vi "Generate NIPKG List.vi"() -> ()   [LabVIEW 2017]
uses:
  <vilib>/National Instruments/NIPM API (Beta)/_support/package attributes.ctl
  <vilib>/National Instruments/NIPM API (Beta)/NIPM_API.lvlib
  NIPKG Support/NIPKG SBOM Support.lvlib
panel:
  in  "stop":bool
  out "Current Package":T1={"Package Name"="", "Display name"="", "Version"="", "Display version"="", "Synopsis"="", "Description"="", "Maintainer"="", "Maintainer email address"="", "Category"="", "Homepage"="", "Release notes"="", "Depends"=[], "Recommends"=[], "Suggests"=[], "Conflicts"=[], "Provides"=[], "Replaces"=[], "Supplements"=[], "Enhances"=[], "Product"=FALSE, "User visible"=FALSE, "Installed size (KB)"=0, "Package filesize (bytes)"=0, "Architecture"="", "Agent"="file", "MD5Checksum"=""}
  out "Installed NI Packages":string[][](table)
  # "Retrieves list of all installed NIPKGs"
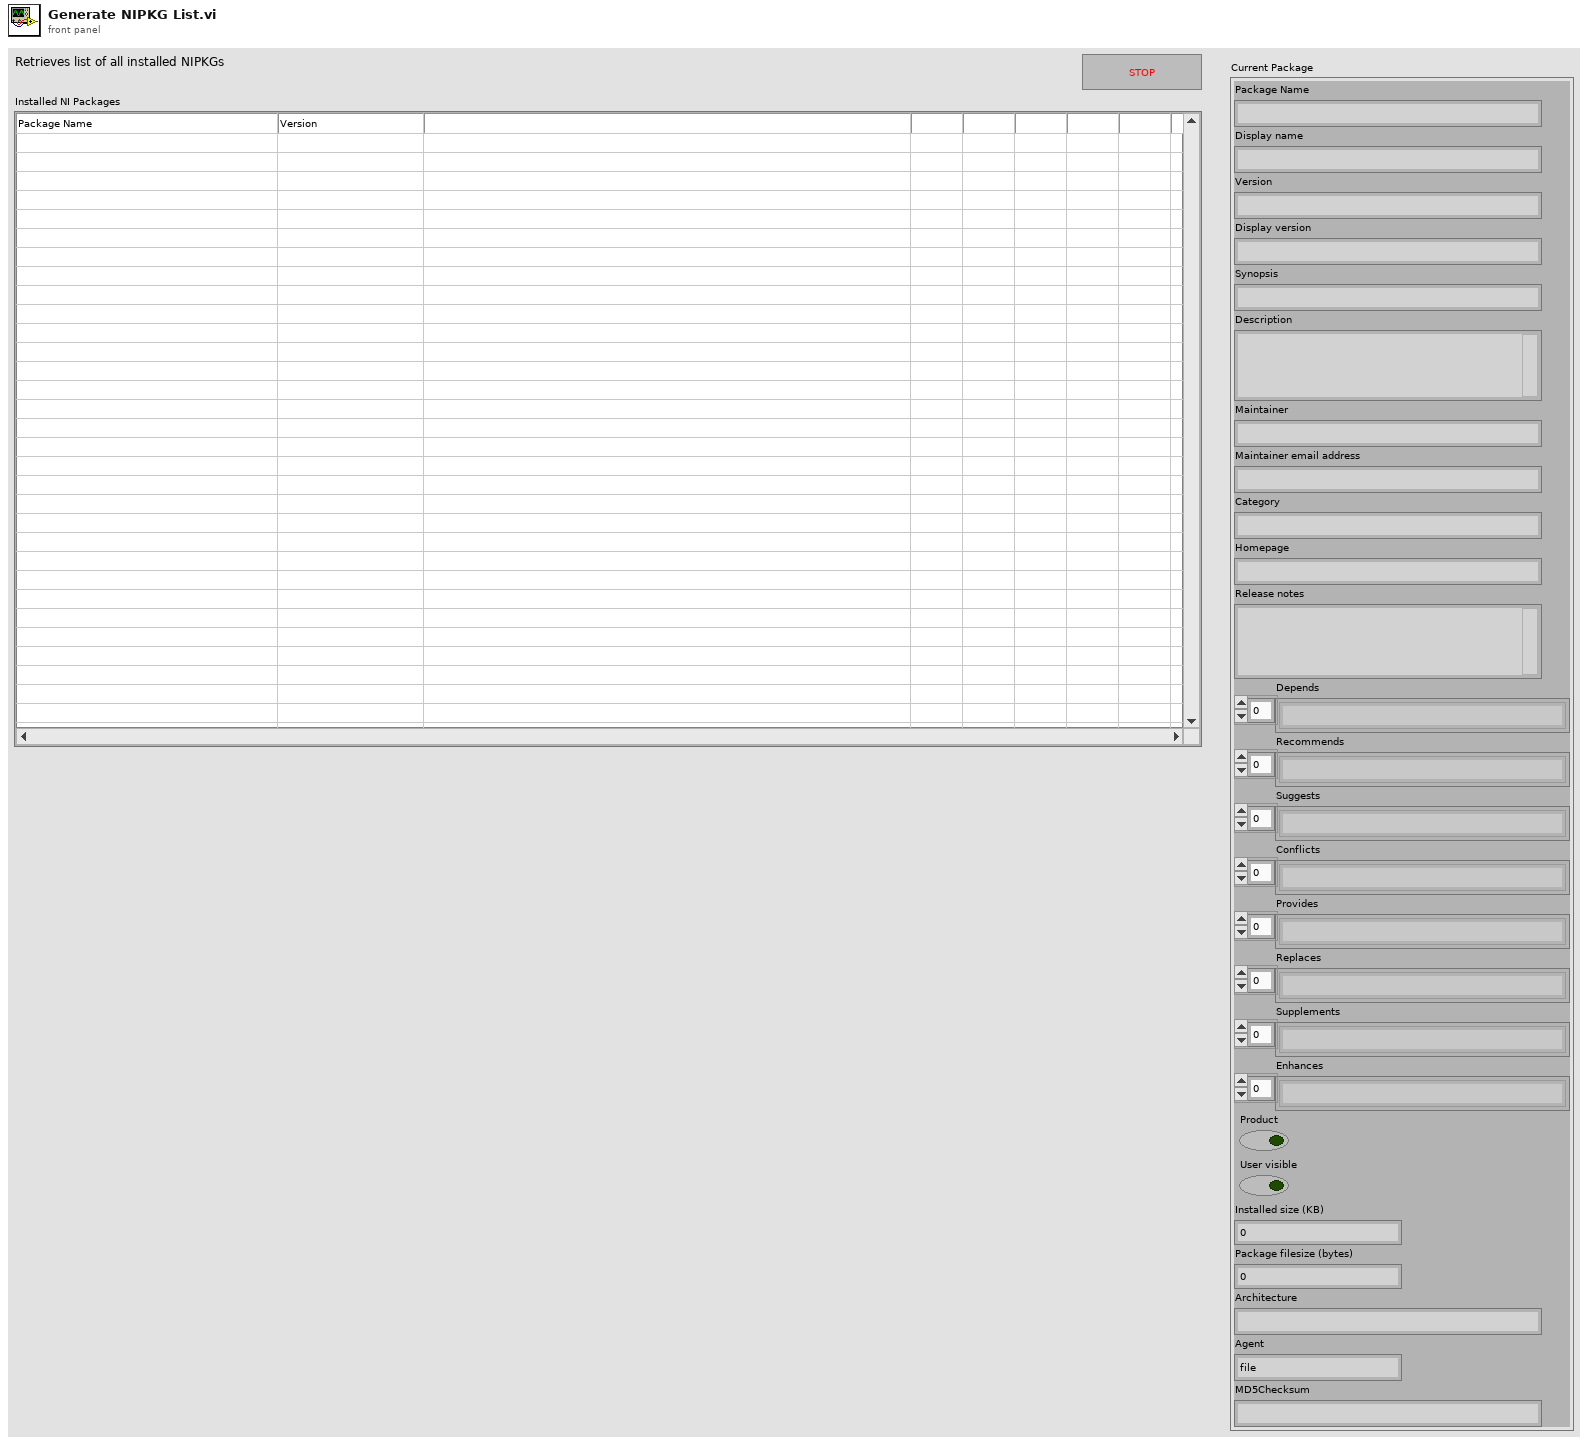
[diagram p1: front panel]
types:
  T1 = typedef "NIPM_API.lvlib/package attributes.ctl" = cluster{"Package Name":string, "Display name":string, "Version":string, "Display version":string, "Synopsis":string, "Description":string, "Maintainer":string, "Maintainer email address":string, "Category":string, "Homepage":string, "Release notes":string, "Depends":string[], "Recommends":string[], "Suggests":string[], "Conflicts":string[], "Provides":string[], "Replaces":string[], "Supplements":string[], "Enhances":string[], "Product":bool, "User visible":bool, "Installed size (KB)":u64, "Package filesize (bytes)":u64, "Architecture":string, "Agent":string, "MD5Checksum":string}
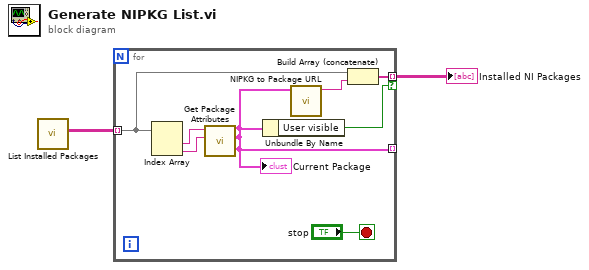
[diagram p0: block diagram]
diagram:
  n1 = call <vilib>:"List Installed Packages.vi"() -> ("installed packages"=w2:string[][])  [unwired: 10 in, 1 out]
  n2 = for {
    tunnel: w2 -> [w7] mode=indexing
    tunnel: [w5] -> w1 mode=indexing if=w4
    tunnel: [w3] -> _ mode=indexing
    stop <- "stop" stop-if-true
    n3 = Index Array(array=w7) -> (element #1=w9:string, element #2=w8:string)  [unwired: 2 in]
    n4 = call <vilib>:"Get Package Attributes.vi"("version"=w8, "package name"=w9) -> ("package attributes"=w3:T1)  [unwired: 6 in, 3 out]
    "Current Package" <- w3
    n5 = Unbundle By Name(w3) -> ("User visible"=w4:bool)
    n6 = call "NIPKG to Package URL.vi"("package attributes"=w3) -> ("NIPKG Package URL"=w6:string)  [unwired: 10 in]
    n7 = Build Array (concatenate)(w7, w6) -> (w5:string[])
  }
  "Installed NI Packages" <- w1
